vi "host.vi"() -> ()   [LabVIEW 2020]
uses:
  <vilib>/FPGAPlugInAG/cRIO-9035/niLvFpga_Open_cRIO-9035.vi
  <vilib>/rvi/interface/common/dynamic/niFpgaDynamicAddResources.vi
  <vilib>/Utility/error.llb/Error Cluster From Error Code.vi
  <vilib>/rvi/interface/common/niFpgaWaitOnOcc.vi
  <vilib>/rvi/errors/niLvFpgaAdjustHostInterfaceError.vi
  <vilib>/FPGAPlugInAG/Dynamic/niLvFpga_Run_Dynamic.vi
  <vilib>/FPGAPlugInAG/Dynamic/niLvFpga_Close_Dynamic.vi
  <vilib>/rvi/interface/nirviOpenFPGA/nirviOpenFPGA.xnode
  FPGA Bitfiles/fftfpgaapplicati_FPGATarget_FFT2_0CJBxAgxp6E.lvbitx
  FFT.vi
  <vilib>/rvi/interface/nirviMethod/nirviMethod.xnode
  <vilib>/rvi/interface/nirviCloseFPGA/nirviCloseFPGA.xnode
  <vilib>/rvi/errors/niLvFpgaMergeErrorWithErrorCode.vi
  <vilib>/FPGAPlugInAG/Dynamic/niLvFpga_ReadFifo_Dynamic.vi
  <vilib>/Analysis/NI_AALPro.lvlib
  <vilib>/FPGAPlugInAG/Dynamic/niLvFpga_ConfigureFifo_Dynamic.vi
  <vilib>/FPGAPlugInAG/Dynamic/niLvFpga_StartFifo_Dynamic.vi
  <vilib>/FPGAPlugInAG/Dynamic/niLvFpga_WriteFifo_Dynamic.vi
panel:
  out "frequency index":dbl[](graph)
  out "frequency size":i32
  out "freq":fxp<+/-,32,15>[](array[numeric])
  out "magnitude":dbl[](graph)
  out "phase":dbl[](graph)
  out "phase size":i32
  out "mag size":i32
  out "phase":fxp<+/-,32,15>[](array[numeric])
  out "magnitude":fxp<+/-,32,15>[](array[numeric])
  out "Actual Depth":u32
  out "host to target":u32
  out "signal_target_to_host_fixed size(s)":i32
  out "target to host 1":u32
  out "signal target to host":dbl[][](graph)
  out "signal_target_to_host_fixed":fxp<+/-,24,7>[](array[numeric])
  out "Array 2":fxp<+/-,24,7>[](array[numeric])
  out "detrend acc":dbl[](graph)
  out "samples":i32
  out "input signal":T1(graph)
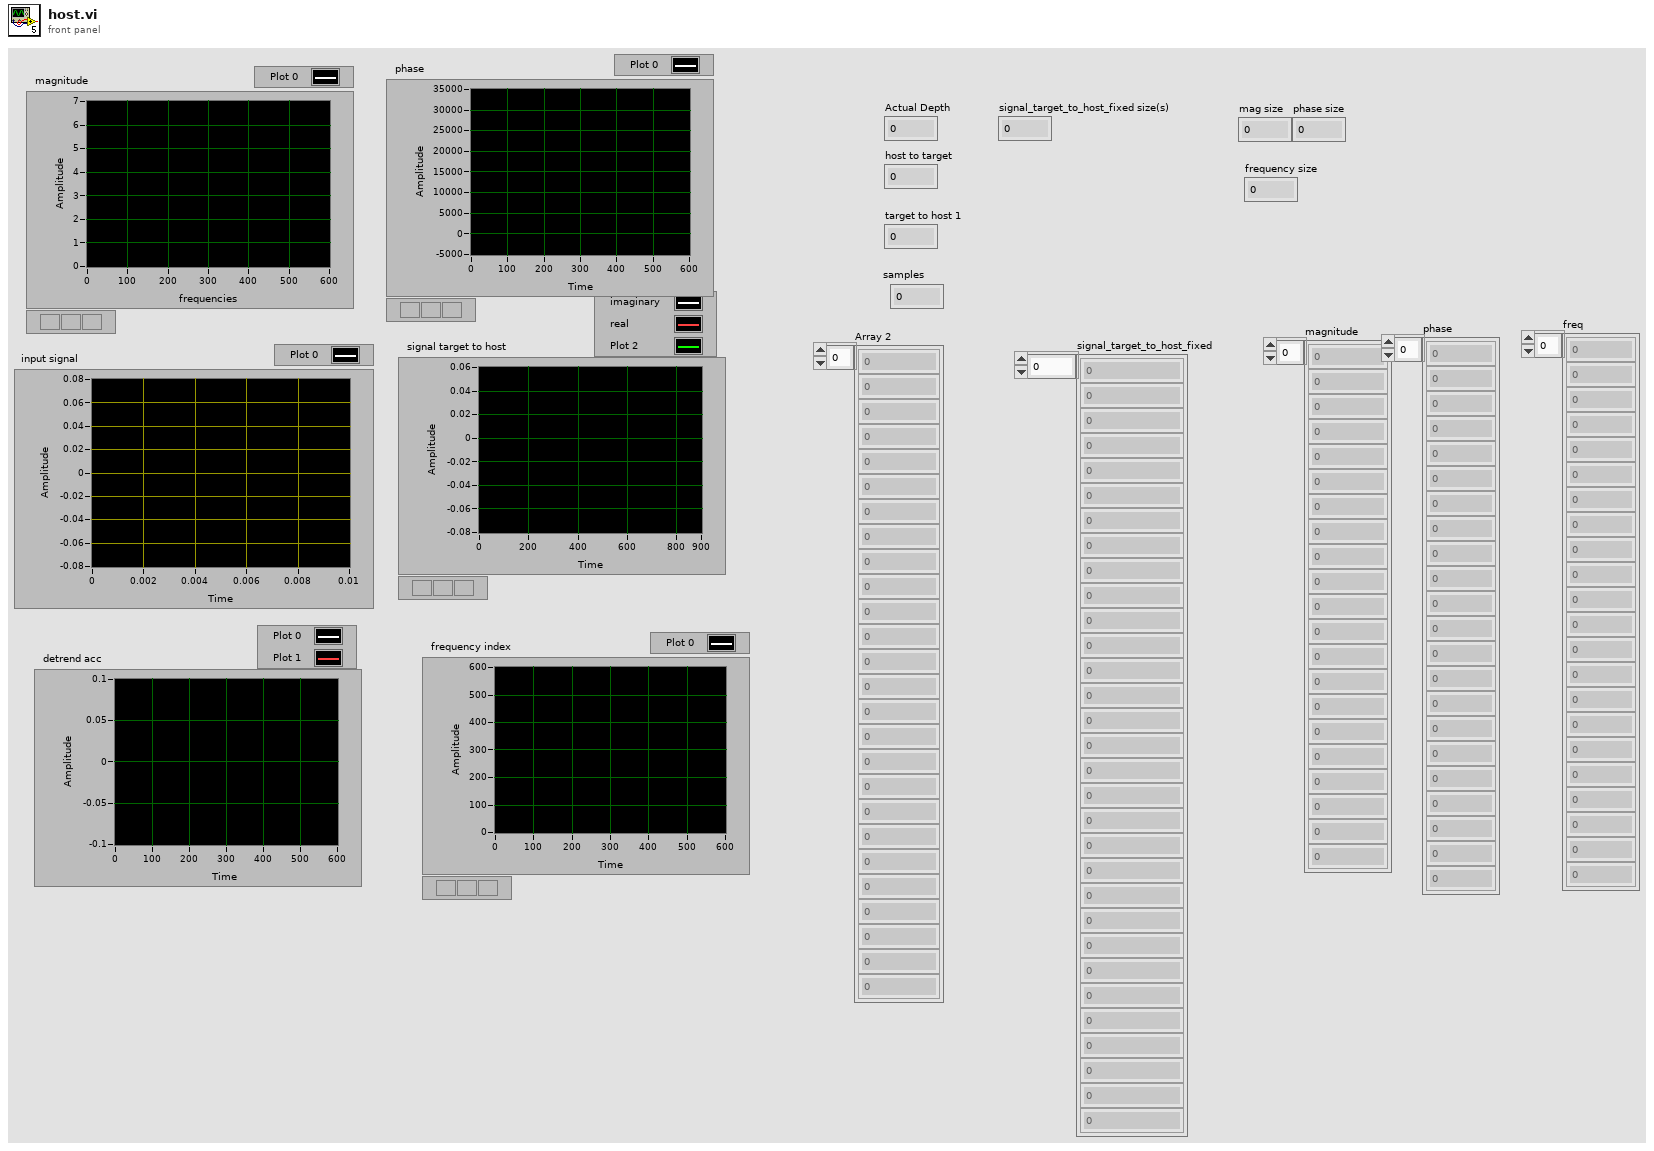
[diagram p1: front panel]
types:
  T1 = cluster{"array type (2D Dbl)":dbl[], "array type (2D Dbl)":dbl[]}
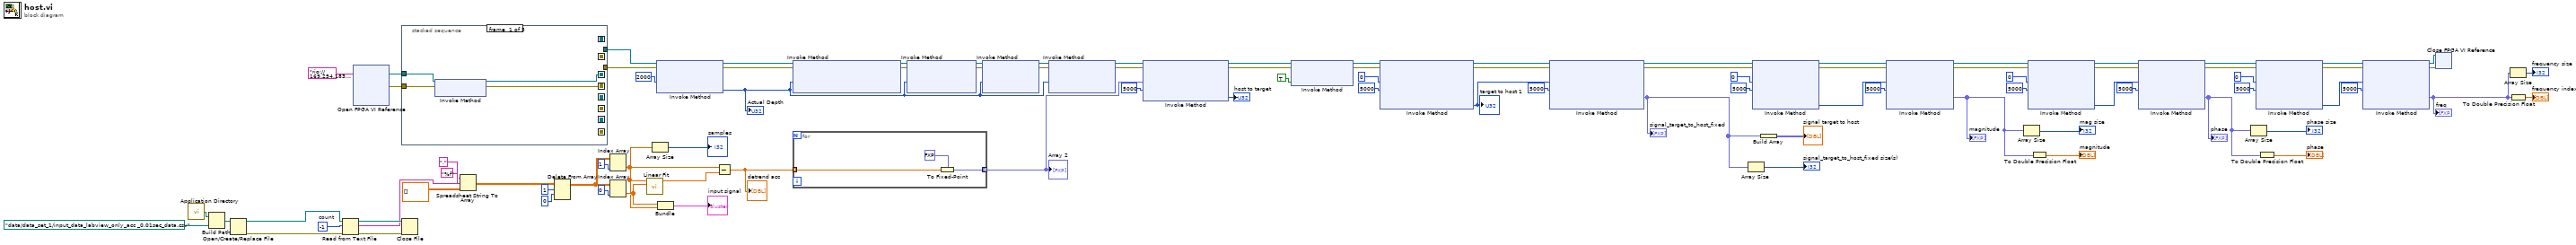
[diagram p0: block diagram]
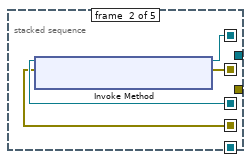
[diagram p2: hidden frame]
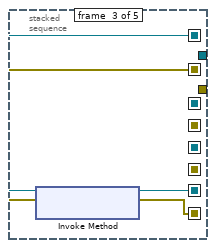
[diagram p3: hidden frame]
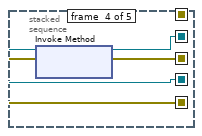
[diagram p4: hidden frame]
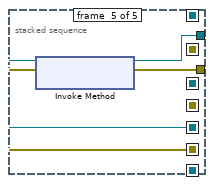
[diagram p5: hidden frame]
diagram:
  w84 = -1  # count
  n1 = call <vilib>:"Application Directory.vi"() -> ("Application Directory"=w88:path)
  n2 = Build Path(base path=w88, name or relative path=path "data/data_set_1/input_data_labview_only_acc _0.01sec_data.csv" ("default name")) -> (appended path=w87:path)
  n3 = Open/Create/Replace File(file path (use dialog)=w87) -> (refnum out=w92:refnum<file>, error out=w93:errorcluster)  [unwired: 5 in, 1 out]
  n4 = Read from Text File(file (use dialog)=w92, count=w84, error in=w93) -> (refnum out=w91:refnum<file>, text=w89:string, error out=w90:errorcluster)  [unwired: 1 in, 1 out]
  n5 = xnode "Open FPGA VI Reference"("resource name"=tag "rio://169.254.183.73/RIO0") -> ("FPGA VI Reference Out"=w51:refnum<k20>, "error out"=w50:errorcluster)  [unwired: 1 in]
  n6 = stacked-sequence {
    seq-local: [w95 _ _ _ _] -> [_ w101 _ _ _]
    seq-local: [w94 _ _ _ _] -> [_ w100 _ _ _]
    seq-local: [_ w99 _ _ _] -> [_ _ w105 _ _]
    seq-local: [_ w98 _ _ _] -> [_ _ w104 _ _]
    seq-local: [_ _ w103 _ _] -> [_ _ _ w109 _]
    seq-local: [_ _ w102 _ _] -> [_ _ _ w108 _]
    seq-local: [_ _ _ w107 _] -> [_ _ _ _ w113]
    seq-local: [_ _ _ w106 _] -> [_ _ _ _ w112]
    tunnel: w51 -> [w97 _ _ _ _]
    tunnel: w50 -> [w96 _ _ _ _]
    tunnel: [_ _ _ _ w111] -> w7
    tunnel: [_ _ _ _ w110] -> w6
    frame #0 {
      n7 = xnode "Invoke Method"("FPGA VI Reference In"=w97, "error in"=w96) -> ("FPGA VI Reference Out"=w95:refnum<k20>, "error out"=w94:errorcluster)
    }
    frame #1 {
      n8 = xnode "Invoke Method"("FPGA VI Reference In"=w101, "error in"=w100) -> ("FPGA VI Reference Out"=w99:refnum<k20>, "error out"=w98:errorcluster)
    }
    frame #2 {
      n9 = xnode "Invoke Method"("FPGA VI Reference In"=w105, "error in"=w104) -> ("FPGA VI Reference Out"=w103:refnum<k20>, "error out"=w102:errorcluster)
    }
    frame #3 {
      n10 = xnode "Invoke Method"("FPGA VI Reference In"=w109, "error in"=w108) -> ("FPGA VI Reference Out"=w107:refnum<k20>, "error out"=w106:errorcluster)
    }
    frame #4 {
      n11 = xnode "Invoke Method"("FPGA VI Reference In"=w113, "error in"=w112) -> ("FPGA VI Reference Out"=w111:refnum<k20>, "error out"=w110:errorcluster)
    }
  }
  n12 = Close File(refnum=w91, error in=w90) -> ()  [unwired: 2 out]
  n13 = Spreadsheet String To Array(delimiter (Tab)=",", format string="%f", spreadsheet string=w89, array type (2D Dbl)=dbl[][] []) -> (array=w81:dbl[][])
  n14 = Delete From Array(array=w81, length=1, index (row)=0) -> (array with subset deleted=w76:dbl[][])  [unwired: 1 in, 1 out]
  n15 = Index Array(array=w76, index (col)=1 ("disabled index (col)")) -> (element=w66:dbl[])  [unwired: 1 in]
  n16 = Index Array(array=w76, index (col)=0 ("disabled index (col)")) -> (element=w68:dbl[])  [unwired: 1 in]
  n17 = call <vilib>:"Linear Fit.vi"("Y"=w66, "X"=w68) -> ("Best Linear Fit"=w67:dbl[])  [unwired: 9 in, 4 out]
  n18 = Array Size(array=w66) -> (size(s)=→"samples":i32)
  n19 = xnode "Invoke Method"("FPGA VI Reference In"=w7, "error in"=w6, "Requested Depth"=u32 2000) -> ("FPGA VI Reference Out"=w49:refnum<k20>, "error out"=w48:errorcluster, "Actual Depth"=w1:u32)
  "Actual Depth" <- w1
  n20 = Bundle("array type (2D Dbl)"=w68, "array type (2D Dbl)"=w66) -> (→"input signal":T1)  [unwired: 1 in]
  n21 = Subtract(x=w66, y=w67) -> (x-y=w65:dbl[])
  "detrend acc" <- w65
  n22 = xnode "Invoke Method"("FPGA VI Reference In"=w49, "error in"=w48, "Requested Depth"=w1) -> ("FPGA VI Reference Out"=w47:refnum<k20>, "error out"=w46:errorcluster)  [unwired: 1 out]
  n23 = for {
    tunnel: [w115] -> w64 mode=indexing
    tunnel: w65 -> [w114] mode=indexing
    n24 = To Fixed-Point(fixed-point type=fxp<+/-,24,7> 0.0 ("f"), number=w114) -> (fixed-point=w115:fxp<+/-,24,7>)
  }
  "Array 2" <- w64
  n25 = xnode "Invoke Method"("FPGA VI Reference In"=w47, "error in"=w46, "Requested Depth"=w1) -> ("FPGA VI Reference Out"=w45:refnum<k20>, "error out"=w44:errorcluster)  [unwired: 1 out]
  n26 = xnode "Invoke Method"("FPGA VI Reference In"=w45, "error in"=w44, "Requested Depth"=w1) -> ("FPGA VI Reference Out"=w5:refnum<k20>, "error out"=w4:errorcluster)  [unwired: 1 out]
  n27 = xnode "Invoke Method"("FPGA VI Reference In"=w5, "error in"=w4, "Requested Depth"=w1) -> ("FPGA VI Reference Out"=w3:refnum<k20>, "error out"=w2:errorcluster)  [unwired: 1 out]
  n28 = xnode "Invoke Method"("FPGA VI Reference In"=w3, "error in"=w2, "Data"=w64, "Timeout (ms)"=5000) -> ("FPGA VI Reference Out"=w73:refnum<k20>, "error out"=w72:errorcluster, "Empty Elements Remaining"=→"host to target":u32)
  n29 = xnode "Invoke Method"("FPGA VI Reference In"=w73, "error in"=w72, "Wait Until Done (F)"=TRUE) -> ("FPGA VI Reference Out"=w55:refnum<k20>, "error out"=w54:errorcluster)
  n30 = xnode "Invoke Method"("FPGA VI Reference In"=w55, "error in"=w54, "Number of Elements"=u32 0, "Timeout (ms)"=5000) -> ("FPGA VI Reference Out"=w63:refnum<k20>, "error out"=w62:errorcluster, "Elements Remaining"=w61:u32)  [unwired: 1 out]
  "target to host 1" <- w61
  n31 = xnode "Invoke Method"("FPGA VI Reference In"=w63, "error in"=w62, "Number of Elements"=w61, "Timeout (ms)"=5000) -> ("FPGA VI Reference Out"=w26:refnum<k20>, "error out"=w25:errorcluster, "Data"=w57:fxp<+/-,24,7>[])  [unwired: 1 out]
  "signal_target_to_host_fixed" <- w57
  n32 = Array Size(array=w57) -> (size(s)=→"signal_target_to_host_fixed size(s)":i32)
  n33 = xnode "Invoke Method"("FPGA VI Reference In"=w26, "error in"=w25, "Number of Elements"=u32 0, "Timeout (ms)"=5000) -> ("FPGA VI Reference Out"=w40:refnum<k20>, "error out"=w39:errorcluster, "Elements Remaining"=w34:u32)  [unwired: 1 out]
  n34 = Build Array(w57) -> (→"signal target to host":fxp<+/-,24,7>[][])
  n35 = xnode "Invoke Method"("FPGA VI Reference In"=w40, "error in"=w39, "Number of Elements"=w34, "Timeout (ms)"=5000) -> ("FPGA VI Reference Out"=w38:refnum<k20>, "error out"=w37:errorcluster, "Data"=w24:fxp<+/-,32,16>[])  [unwired: 1 out]
  "magnitude" <- w24
  n36 = Array Size(array=w24) -> (size(s)=→"mag size":i32)
  n37 = xnode "Invoke Method"("FPGA VI Reference In"=w38, "error in"=w37, "Number of Elements"=u32 0, "Timeout (ms)"=5000) -> ("FPGA VI Reference Out"=w36:refnum<k20>, "error out"=w35:errorcluster, "Elements Remaining"=w30:u32)  [unwired: 1 out]
  n38 = To Double Precision Float(number=w24) -> (double precision float=→"magnitude":dbl[])
  n39 = xnode "Invoke Method"("FPGA VI Reference In"=w36, "error in"=w35, "Number of Elements"=w30, "Timeout (ms)"=5000) -> ("FPGA VI Reference Out"=w11:refnum<k20>, "error out"=w10:errorcluster, "Data"=w23:fxp<+/-,32,16>[])  [unwired: 1 out]
  "phase" <- w23
  n40 = Array Size(array=w23) -> (size(s)=→"phase size":i32)
  n41 = xnode "Invoke Method"("FPGA VI Reference In"=w11, "error in"=w10, "Number of Elements"=u32 0, "Timeout (ms)"=5000) -> ("FPGA VI Reference Out"=w20:refnum<k20>, "error out"=w19:errorcluster, "Elements Remaining"=w16:u32)  [unwired: 1 out]
  n42 = To Double Precision Float(number=w23) -> (double precision float=→"phase":dbl[])
  n43 = xnode "Invoke Method"("FPGA VI Reference In"=w20, "error in"=w19, "Number of Elements"=w16, "Timeout (ms)"=5000) -> ("FPGA VI Reference Out"=w9:refnum<k20>, "error out"=w8:errorcluster, "Data"=w13:fxp<+/-,32,16>[])  [unwired: 1 out]
  "freq" <- w13
  n44 = xnode "Close FPGA VI Reference"("FPGA VI Reference In"=w9, "error in"=w8) -> ()  [unwired: 1 out]
  n45 = Array Size(array=w13) -> (size(s)=→"frequency size":i32)
  n46 = To Double Precision Float(number=w13) -> (double precision float=→"frequency index":dbl[])
